vi "CD Read Engine_Retrieve Records.vi"(8 "error in (no error)":errorcluster, 9 "bytes read":i32, 11 "core reader handle in":u64) -> (0 "error out":errorcluster, 1 "# of records read":i32, 3 "Array of Records":T1[](array[typedef]) {"type" format="%04x"; "activity" format="%04x"; "error" format="%04x"; "cwd1" format="%04x"; "cwd2" format="%04x"; "swd1" format="%04x"; "swd2" format="%04x"; "data" format="%04x"})   [LabVIEW 2017, in "Ballard MIL-1553 Engine.lvlib"]
uses:
  Ballard MIL-1553 Engine.lvlib
  <instrlib>/BTICardLib/Public/Controls/1553 Record.ctl
  <instrlib>/BTICardLib/BTICardLV.lvlib
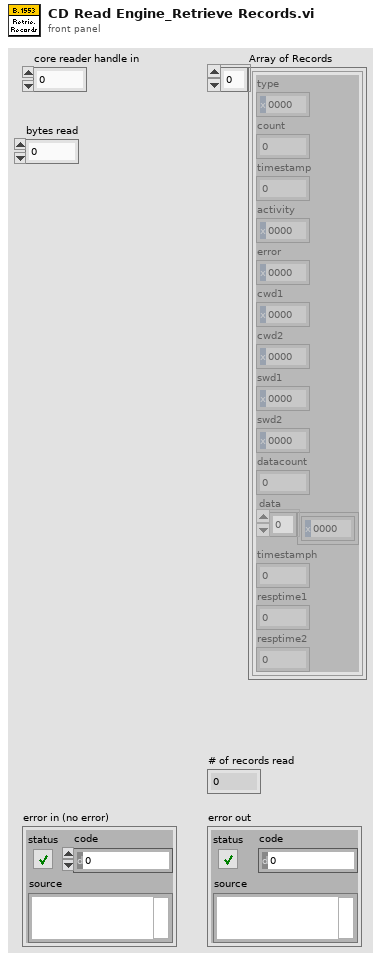
[diagram p1: front panel]
types:
  T1 = typedef "BTICardLV.lvlib/1553 Record.ctl" = cluster{"type":u16, "count":u16, "timestamp":u32, "activity":u16, "error":u16, "cwd1":u16, "cwd2":u16, "swd1":u16, "swd2":u16, "datacount":u16, "data":u16[], "timestamph":u32, "resptime1":u16, "resptime2":u16}
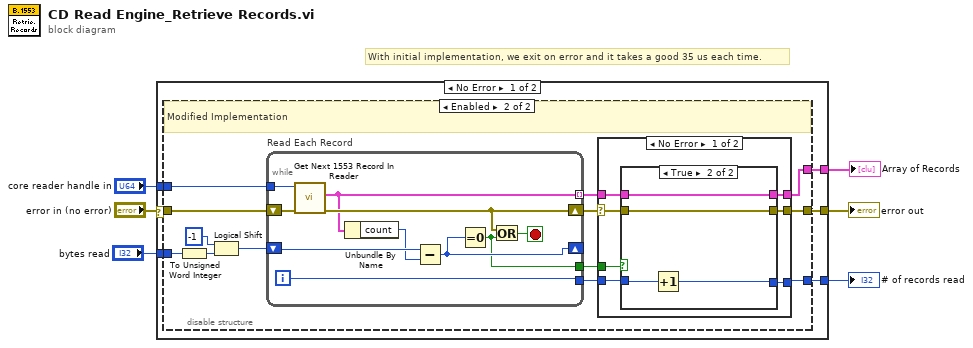
[diagram p0: block diagram]
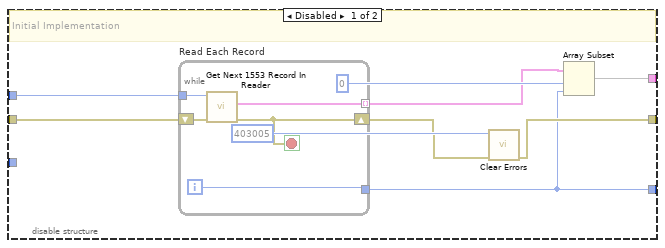
[diagram p2: hidden frame]
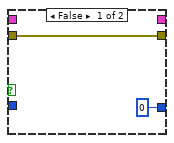
[diagram p3: hidden frame]
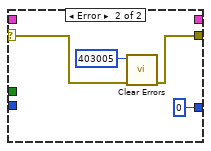
[diagram p4: hidden frame]
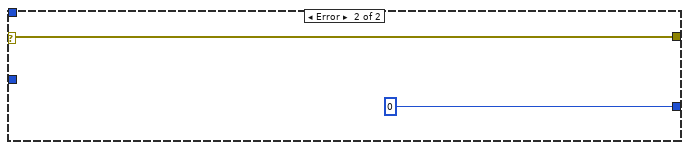
[diagram p5: hidden frame]
diagram:
  # "With initial implementation, we exit on error and it takes a good 35 us each time."
  n1 = case shown="No Error" "error in (no error)" {
    selector: "error in (no error)" -> [w8 w68]
    tunnel: "core reader handle in" -> [w12 _]
    tunnel: [w11 w68] -> w5
    tunnel: [w10 _] -> w4
    tunnel: [w9 0] -> w3
    tunnel: "bytes read" -> [w7 _]
    frame No Error {
      n2 = disable-structure shown="Enabled" {
        disable-tunnel: w12 -> [w21 w39]
        disable-tunnel: [w18 w27] -> w11
        disable-tunnel: [w15 w28] -> w10
        disable-tunnel: [w14 w29] -> w9
        disable-tunnel: w8 -> [w13 w36]
        disable-tunnel: w7 -> [_ w35]
        frame Disabled {
          # "Initial Implementation"
          n3 = while "Read Each Record" {
            tunnel: w21 -> [w26]
            tunnel: [w23] -> w16 mode=indexing
            shift-right: [w24] -> w19
            shift-left: w13 -> [w25]
            tunnel: [w22] -> w14
            i -> [w22]
            stop <- w24 stop-if-true
            n4 = call <instrlib>:"Get Next 1553 Record In Reader.vi"("error in (no error)"=w25, "core reader handle in"=w26) -> ("error out"=w24:errorcluster, "record out"=w23:T1)  [unwired: 7 in, 1 out]
          }
          n5 = call <vilib>:"Clear Errors.vi"("error in (no error)"=w19, "specific error code to clear (0: all)"=403005) -> ("error out"=w18:errorcluster)  [unwired: 4 in, 1 out]
          n6 = Array Subset(array=w16, index=0, length=w14) -> (w15:T1[])
        }
        frame Enabled {
          # "Modified Implementation"
          n7 = To Unsigned Word Integer(number=w35) -> (unsigned 16bit integer=w32:u16)
          n8 = Logical Shift(y=i16 -1, x=w32) -> (x << y=w33:u16)
          n9 = while "Read Each Record" {
            tunnel: w39 -> [w66]
            tunnel: [w62] -> w38 mode=indexing
            shift-right: [w63] -> w31
            shift-left: w36 -> [w65]
            tunnel: [w64] -> w37
            shift-right: [w59] -> _
            shift-left: w33 -> [w61]
            tunnel: [w58] -> w30
            i -> [w64]
            stop <- w57 stop-if-true
            n10 = call <instrlib>:"Get Next 1553 Record In Reader.vi"("error in (no error)"=w65, "core reader handle in"=w66) -> ("error out"=w63:errorcluster, "record out"=w62:T1)  [unwired: 7 in, 1 out]
            n11 = Unbundle By Name(w62) -> ("count"=w60:u16)
            n12 = Subtract(x=w61, y=w60) -> (x-y=w59:u16)
            n13 = Equal To 0?(x=w59) -> (x = 0?=w58:bool)
            n14 = Or(x=w63, y=w58) -> (x .or. y?=w57:bool)
          }
          n15 = case shown="No Error" w31 {
            selector: w31 -> [w43 w55]
            tunnel: w38 -> [w42 _]
            tunnel: w37 -> [w45 _]
            tunnel: w30 -> [w46 _]
            tunnel: [w44 0] -> w29
            tunnel: [w41 _] -> w28
            tunnel: [w40 w54] -> w27
            frame No Error {
              n16 = case shown="True" w46 {
                tunnel: w45 -> [_ w52]
                tunnel: [0 w51] -> w44
                tunnel: w43 -> [w47 w49]
                tunnel: w42 -> [_ w50]
                tunnel: [_ w50] -> w41
                tunnel: [w47 w49] -> w40
                frame False {
                }
                frame True {
                  n17 = Increment(x=w52) -> (x+1=w51:i32)
                }
              }
            }
            frame Error {
              n18 = call <vilib>:"Clear Errors.vi"("error in (no error)"=w55, "specific error code to clear (0: all)"=403005) -> ("error out"=w54:errorcluster)  [unwired: 4 in, 1 out]
            }
          }
        }
      }
    }
    frame Error {
    }
  }
  "Array of Records" <- w4
  "error out" <- w5
  "# of records read" <- w3
